vi "Controller.vi"(7 "Controller":T1={"Control Algorithm selector"=enum."LQG-LTR", "K"={"A"=[[-4.94989, 0.0218181, -352.966, 23.8192, -3.10685, -0.000952287], [-0.0218181, -4.904857, 23.4819, -343.472, 0.000977323, -3.58066], [0.0389045, 0.0, -31.6573, 0.0287797, 0.0245405, 0.0], [0.0, 0.0381972, 0.0287797, -31.6573, 0.0, 0.0280468], [0.0, 0.0325383, 0.0240248, -0.0293675, -0.0245405, 0.0], [0.031831, 0.0, -0.0282058, 0.0, 0.0, 0.0]], "B"=[[28.0692, -23.9099], [-23.3912, 28.5852], [31.6468, -0.0287797], [-0.0287797, 31.6468], [-0.0282058, -0.0293675], [0.0282058, -0.0240214]], "C"=[[4.94989, 0.0218181, 314.896, 0.0907351, 3.10685, 0.000952287], [10.0218181, 4.90457, -0.0906726, 314.884, -0.000977323, 3.58066]], "D"=[[0.0, 0.0], [0.0, 0.0]]}, "PI"={"A"=[[-4.94989, 0.0218181, -352.966, 23.8192, -3.10685, -0.000952287], [-0.0218181, -4.904857, 23.4819, -343.472, 0.000977323, -3.58066], [0.0389045, 0.0, -31.6573, 0.0287797, 0.0245405, 0.0], [0.0, 0.0381972, 0.0287797, -31.6573, 0.0, 0.0280468], [0.0, 0.0325383, 0.0240248, -0.0293675, -0.0245405, 0.0], [0.031831, 0.0, -0.0282058, 0.0, 0.0, 0.0]], "B"=[[28.0692, -23.9099], [-23.3912, 28.5852], [31.6468, -0.0287797], [-0.0287797, 31.6468], [-0.0282058, -0.0293675], [0.0282058, -0.0240214]], "C"=[[4.94989, 0.0218181, 314.896, 0.0907351, 3.10685, 0.000952287], [10.0218181, 4.90457, -0.0906726, 314.884, -0.000977323, 3.58066]], "D"=[[0.0, 0.0], [0.0, 0.0]]}}, 8 "error in (no error)":errorcluster, 10 "Tanks levels":dbl[](array[numeric]), 11 "Setpoints":T3) -> (0 "error out":errorcluster, 2 "Pumps Voltages":dbl[](array[numeric]), 5 "Plant Control Variables":T4)   [LabVIEW 2018]
uses:
  <vilib>/Simulation/Implementation/XNodeFramework/SimXNode/SimX.xnode
  <vilib>/Simulation/DiscreteLinear/Implementation/NILVSim Discrete State Space Direct.llb/SIM Discrete State Space Direct Diagram (MIMO).vi
  Control Algorithm Selection.ctl
  Control Algorithm Data.ctl
panel:
  out "Saturated?":bool[](array[boolean])
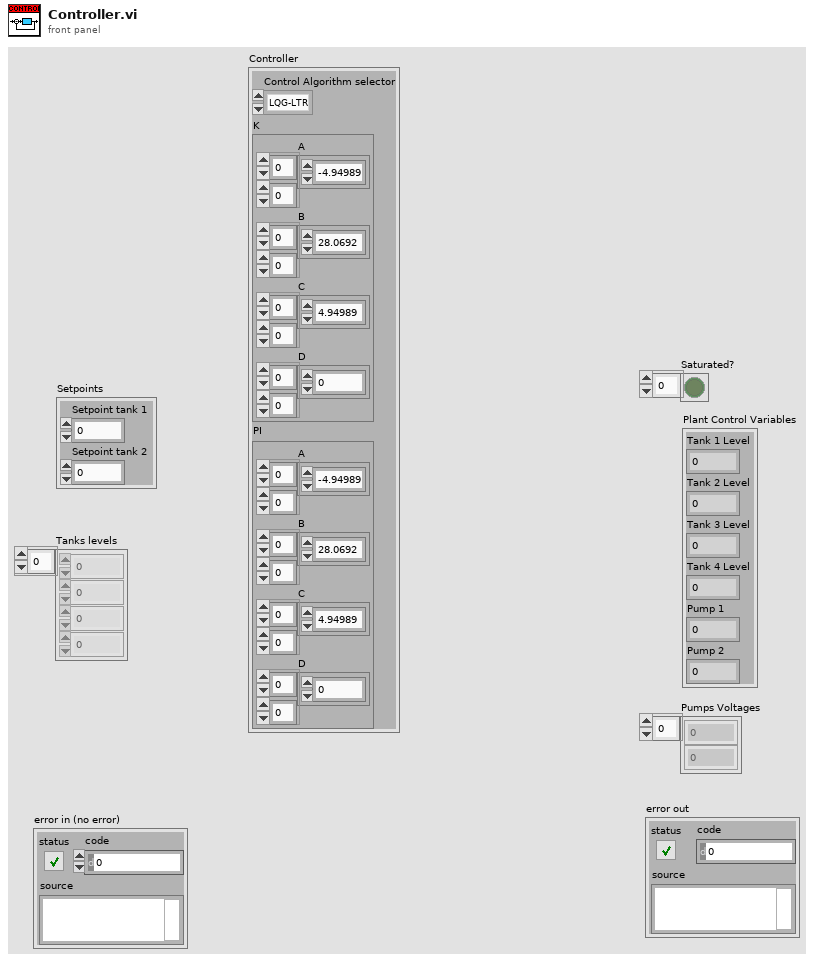
[diagram p1: front panel]
types:
  T1 = typedef "Control Algorithm Data.ctl" = cluster{"Control Algorithm selector":T2, "K":cluster{"A":dbl[][], "B":dbl[][], "C":dbl[][], "D":dbl[][]}, "PI":cluster{"A":dbl[][], "B":dbl[][], "C":dbl[][], "D":dbl[][]}}
  T2 = typedef "Control Algorithm Selection.ctl" = enum16{"LQG-LTR", "Hinf"}
  T3 = cluster{"Setpoint tank 1":dbl, "Setpoint tank 2":dbl}
  T4 = cluster{"Tank 1 Level":dbl, "Tank 2 Level":dbl, "Tank 3 Level":dbl, "Tank 4 Level":dbl, "Pump 1":dbl, "Pump 2":dbl}
  T5 = cluster{"A":dbl[][], "B":dbl[][], "C":dbl[][], "D":dbl[][]}
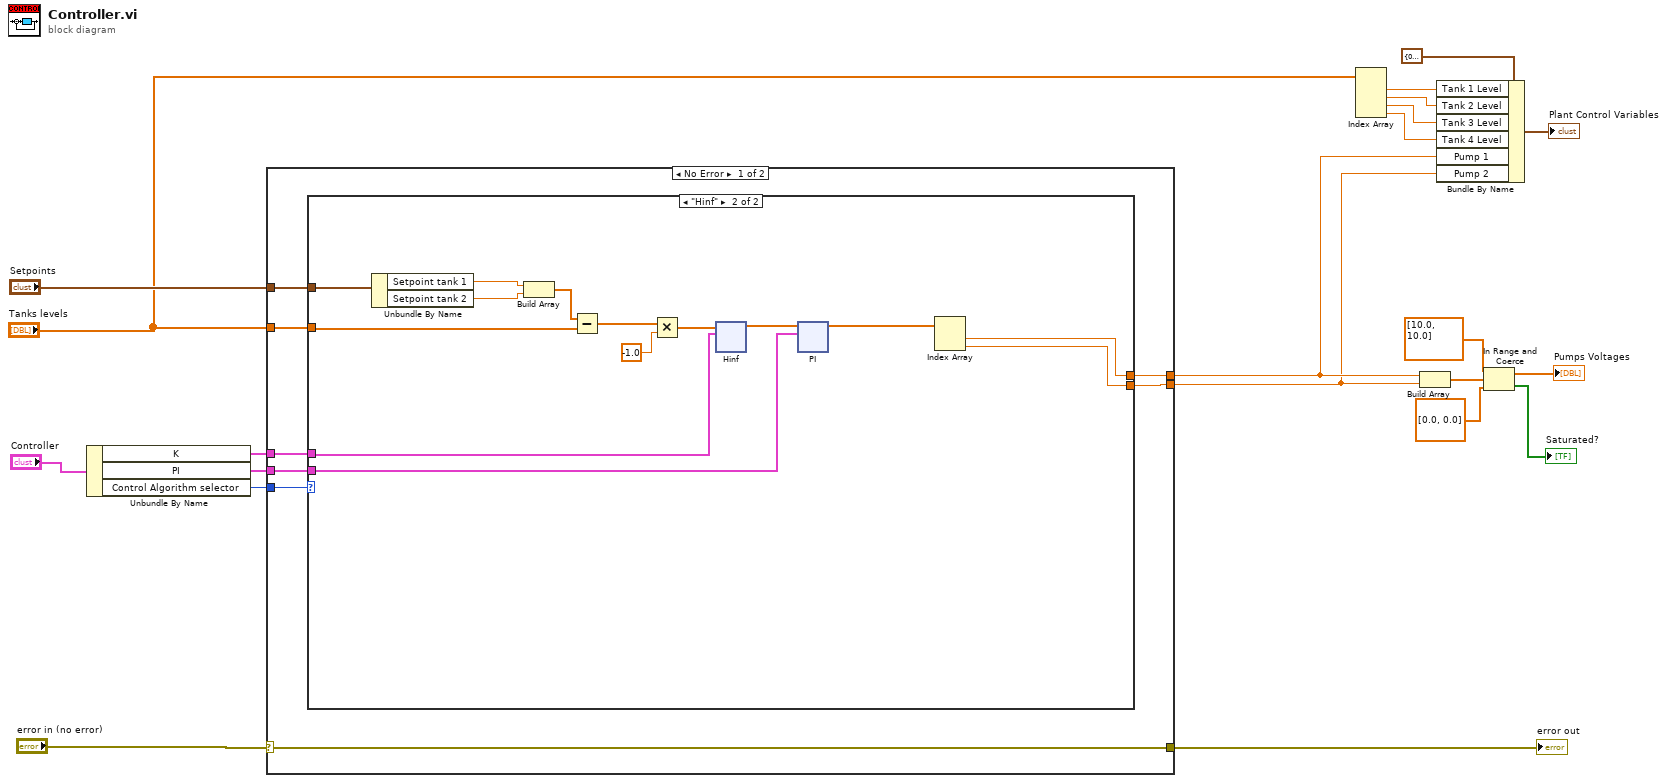
[diagram p0: block diagram]
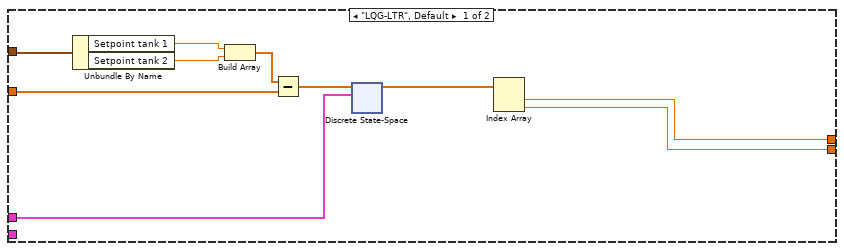
[diagram p2: hidden frame]
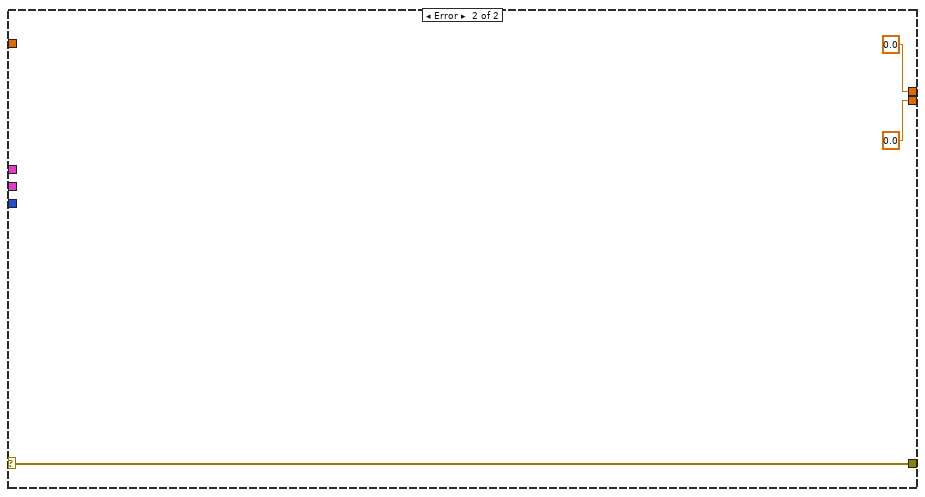
[diagram p3: hidden frame]
diagram:
  n1 = Unbundle By Name("Controller") -> ("K"=w2:T5, "PI"=w3:T5, "Control Algorithm selector"=w1:T2)
  n2 = case shown="No Error" "error in (no error)" {
    selector: "error in (no error)" -> [w27 w80]
    tunnel: "Setpoints" -> [w29 _]
    tunnel: "Tanks levels" -> [w28 _]
    tunnel: [w25 0.0 ("u1")] -> w13
    tunnel: [w24 0.0 ("u2")] -> w12
    tunnel: [w27 w80] -> w5
    tunnel: w3 -> [w22 _]
    tunnel: w2 -> [w26 _]
    tunnel: w1 -> [w23 _]
    frame No Error {
      n3 = case shown="\"Hinf\"" w23 {
        tunnel: w29 -> [w39 w48]
        tunnel: w28 -> [w35 w58]
        tunnel: w26 -> [w30 w57]
        tunnel: [w32 w56] -> w25
        tunnel: [w31 w55] -> w24
        tunnel: w22 -> [_ w49]
        frame "LQG-LTR", Default {
          n4 = Unbundle By Name(w39) -> ("Setpoint tank 1"=w36:dbl, "Setpoint tank 2"=w37:dbl)
          n5 = Build Array(w36, w37) -> (w38:dbl[])
          n6 = Subtract(x=w38, y=w35) -> (x-y=w34:dbl[])
          n7 = xnode "Discrete State-Space"("input u(k)"=w34, "State-Space"=w30) -> ("output y(k)"=w33:dbl[])  [unwired: 2 in, 3 out]
          n8 = Index Array(array=w33) -> (element #1=w32:dbl, element #2=w31:dbl)  [unwired: 2 in]
        }
        frame "Hinf" {
          n9 = Unbundle By Name(w48) -> ("Setpoint tank 1"=w59:dbl, "Setpoint tank 2"=w60:dbl)
          n10 = Build Array(w59, w60) -> (w61:dbl[])
          n11 = Subtract(x=w61, y=w58) -> (x-y=w54:dbl[])
          n12 = Multiply(x=w54, y=-1.0) -> (x*y=w53:dbl[])
          n13 = xnode "Hinf"("input u(k)"=w53, "State-Space"=w57) -> ("output y(k)"=w51:dbl[])  [unwired: 2 in, 3 out]
          n14 = xnode "PI"("input u(k)"=w51, "State-Space"=w49) -> ("output y(k)"=w50:dbl[])  [unwired: 2 in, 3 out]
          n15 = Index Array(array=w50) -> (element #1=w56:dbl, element #2=w55:dbl)  [unwired: 2 in]
        }
      }
    }
    frame Error {
    }
  }
  "error out" <- w5
  n16 = Index Array(array="Tanks levels") -> (element #1=w19:dbl, element #2=w18:dbl, element #3=w17:dbl, element #4=w16:dbl)  [unwired: 4 in]
  n17 = Build Array(w13, w12) -> (w11:dbl[])
  n18 = Bundle By Name(cluster=T4 {"Tank 1 Level"=0.0, "Tank 2 Level"=0.0, "Tank 3 Level"=0.0, "Tank 4 Level"=0.0, "Pump 1"=0.0, "Pump 2"=0.0} ("Plant Control Variables"), "Tank 1 Level"=w19, "Tank 2 Level"=w18, "Tank 3 Level"=w17, "Tank 4 Level"=w16, "Pump 1"=w13, "Pump 2"=w12) -> (→"Plant Control Variables":T4)
  n19 = In Range and Coerce(upper limit=dbl[] [10.0, 10.0] ("lower limit"), x=w11, lower limit=dbl[] [0.0, 0.0]) -> (coerced(x)=→"Pumps Voltages":dbl[], In Range?=→"Saturated?":bool[])
